vi "Message Path.vi"(9 "Message Method":string, 10 "Class Path":path) -> (2 "Message Class Path":path)   [LabVIEW 2023, in "Message Maker.lvclass"]
doc: "Builds the new message's path\n\nAuthor: Derek Trepanier\nCopyright: MGI 2015"
uses:
  Message Maker.lvclass
  Message Maker.lvclass/Message Maker.ctl
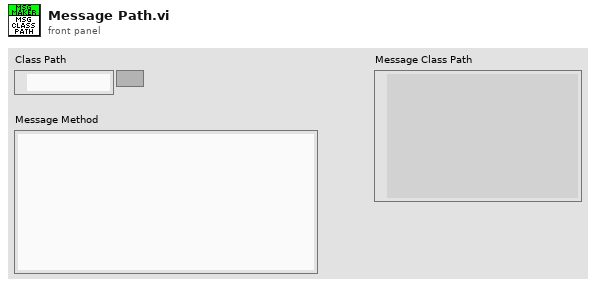
[diagram p1: front panel]
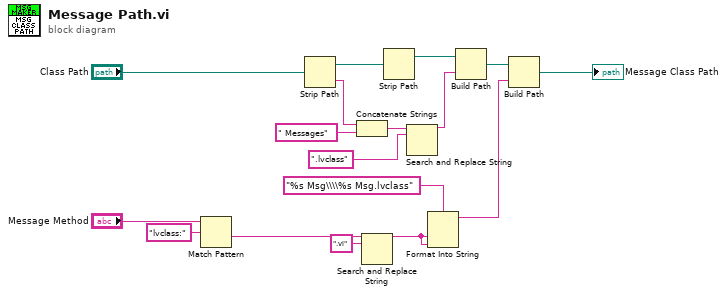
[diagram p0: block diagram]
diagram:
  n1 = Match Pattern(string="Message Method", regular expression="lvclass:") -> (after substring=w1:string)  [unwired: 1 in, 3 out]
  n2 = Strip Path(path="Class Path") -> (stripped path=w10:path, name=w13:string)
  n3 = Concatenate Strings(w13, " Messages" ("string")) -> (w15:string)
  n4 = Search and Replace String(input string=w1, search string=".vi") -> (result string=w6:string)  [unwired: 6 in, 3 out]
  n5 = Strip Path(path=w10) -> (stripped path=w12:path)  [unwired: 1 out]
  n6 = Search and Replace String(input string=w15, search string=".lvclass" ("string")) -> (result string=w16:string)  [unwired: 6 in, 3 out]
  n7 = Format Into String(format string="%s Msg\\\\%s Msg.lvclass", w6, w6) -> (resulting string=w8:string)  [unwired: 2 in, 1 out]
  n8 = Build Path(base path=w12, name or relative path=w16) -> (appended path=w11:path)
  n9 = Build Path(base path=w11, name or relative path=w8) -> (appended path=→"Message Class Path":path)
